vi "Rename.vi"() -> ()   [LabVIEW 2021]
uses:
  <vilib>/Utility/EditLVLibs/Edit LVLibs.lvlib
  _Rename/_Rename.lvlib
panel:
  in  "Name":string="Template"
  in  "Rename":bool
  in  "Rename":string="NEW"
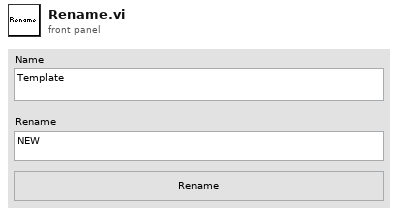
[diagram p1: front panel]
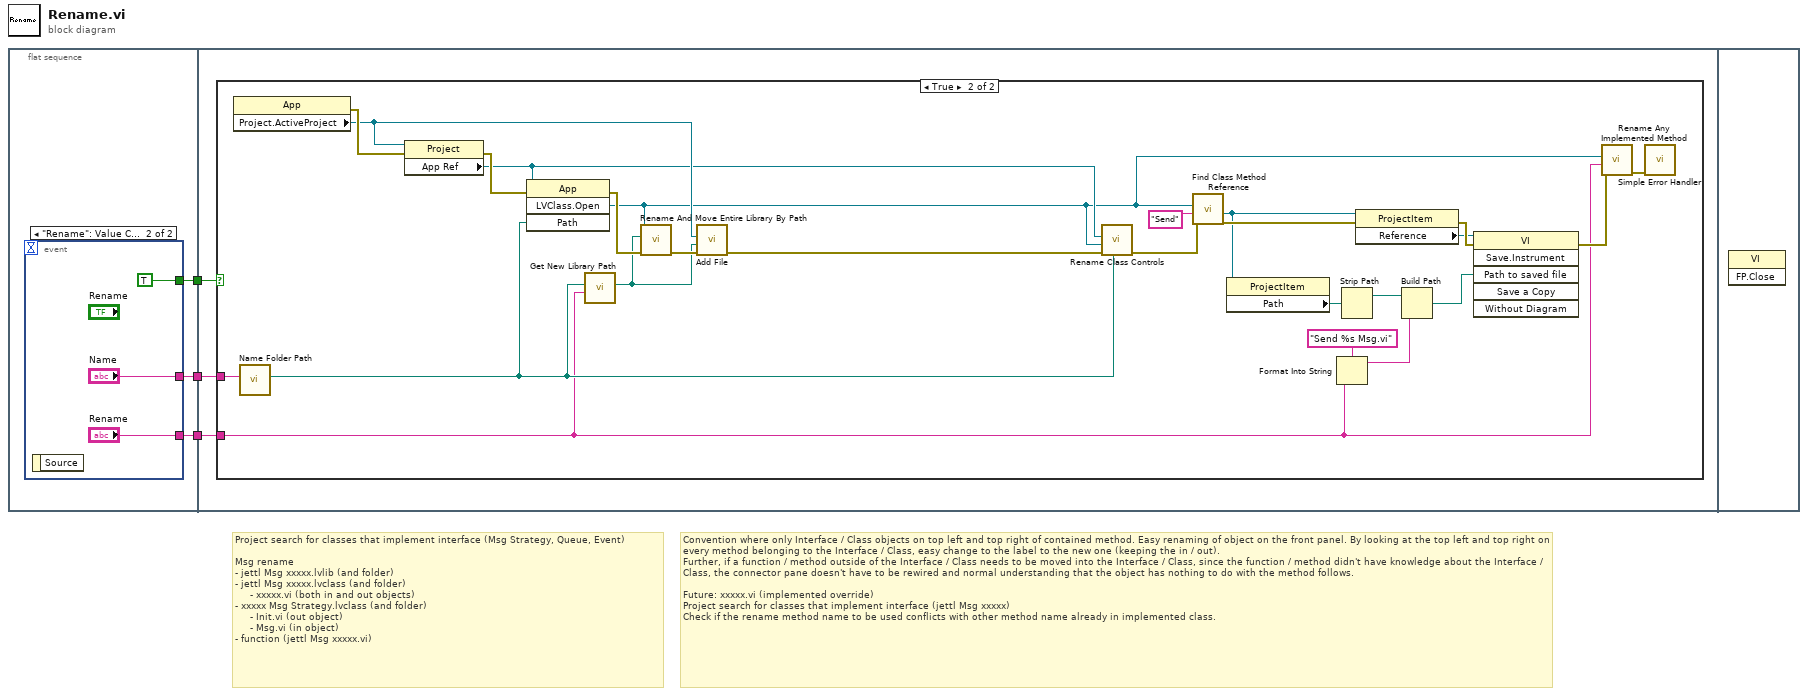
[diagram p0: block diagram]
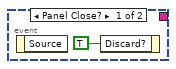
[diagram p2: hidden frame]
diagram:
  # "Convention where only Interface / Class objects on top left and top right of contained method. Easy renaming of object on the front panel. By looking at the top left and top right on every method belonging to the Interface / Class, easy change to the label to the new one (keeping the in / out).\nFurther, if a function / method outside of the Interface / Class needs to be moved into the Interface / Class, since the function / method didn't have knowledge about the Interface / Class, the connector pane doesn't have to be rewired and normal understanding that the object has nothing to do with the method follows.\n\nFuture: xxxxx.vi (implemented override)\nProject search for classes that implement interface (jettl Msg xxxxx)\nCheck if the rename method name to be used conflicts with other method name already in implemented class."
  # "Project search for classes that implement interface (Msg Strategy, Queue, Event)\n\nMsg rename\n- jettl Msg xxxxx.lvlib (and folder)\n- jettl Msg xxxxx.lvclass (and folder)\n     - xxxxx.vi (both in and out objects)\n- xxxxx Msg Strategy.lvclass (and folder)\n     - Init.vi (out object)\n     - Msg.vi (in object)\n- function (jettl Msg xxxxx.vi)"
  n1 = flat-sequence {
    tunnel: [w6] -> w3
    tunnel: [w5] -> w2
    tunnel: [w4] -> w1
    tunnel: w3 -> [w13]
    tunnel: w2 -> [w12]
    tunnel: w1 -> [w11]
    frame #0 {
      n2 = event shown="[1] \"Rename\": Value Change" {
        selector: _ -> [_ _]
        dyn-events: _ -> [_ _]
        timeout: _ -> [_ _]
        tunnel: [_ TRUE ("Rename 2")] -> w6
        tunnel: [_ "Rename"] -> w5
        tunnel: [_ "Name"] -> w4
        event Panel Close? {
          n3 = event-data() -> ()  [unwired: 1 in, 1 out]
          n4 = event-data("Discard?"=TRUE) -> ()  [unwired: 1 in, 1 out]
        }
        event "Rename": Value Change {
          n5 = event-data() -> ()  [unwired: 1 in, 1 out]
        }
      }
    }
    frame #1 {
      n6 = case shown="True" w13 {
        tunnel: w12 -> [_ w17]
        tunnel: w11 -> [_ w19]
        frame False {
        }
        frame True {
          n7 = property class="App"() -> (error out=w37:errorcluster, "Project.ActiveProject"=w21:refnum<vi>)  [unwired: 2 in, 1 out]
          n8 = call "Name Folder Path.vi"("Name"=w19) -> ("Name Folder Path"=w18:path)  [unwired: 10 in]
          n9 = property class="Project"(reference=w21, error in=w37) -> (error out=w35:errorcluster, "App Ref"=w20:refnum<vi>)  [unwired: 1 out]
          n10 = invoke class="App" method="LVClass.Open"(reference=w20, error in=w35, "Path"=w18) -> (error out=w36:errorcluster, "LVClass.Open"=w15:refnum<vi>)  [unwired: 1 in, 2 out]
          n11 = call "Get New Library Path.vi"("Rename"=w17, "Name Folder Path"=w18) -> ("New Library Path"=w16:path)  [unwired: 9 in]
          n12 = call <vilib>:"Rename And Move Entire Library By Path.vi"("error in (no error)"=w36, "New library path"=w16, "Library ref in"=w15) -> ("error out"=w22:errorcluster)  [unwired: 7 in, 1 out]
          n13 = call "Add File.vi"("error in"=w22, "Path"=w16, "Project:Active Project"=w21) -> ("error out"=w14:errorcluster)  [unwired: 8 in]
          n14 = call "Rename Class Controls.vi"("Old Class"=w18, "error in"=w14, "Class To Rename"=w15, "Application Instance"=w20) -> ("error out"=w27:errorcluster)  [unwired: 7 in]
          n15 = call "Find Class Method Reference.vi"("error in"=w27, "Method Name"="Send" ("regular expression"), "Class To Rename"=w15) -> ("error out"=w26:errorcluster, "Method Reference"=w23:refnum<vi>)  [unwired: 7 in]
          n16 = property class="ProjectItem"(reference=w23) -> ("Path"=w29:path)  [unwired: 1 in, 2 out]
          n17 = Format Into String(format string="Send %s Msg.vi", w17) -> (resulting string=w24:string)  [unwired: 2 in, 1 out]
          n18 = Strip Path(path=w29) -> (stripped path=w34:path)  [unwired: 1 out]
          n19 = property class="ProjectItem"(reference=w23, error in=w26) -> (error out=w38:errorcluster, "Reference"=w33:refnum<vi>)  [unwired: 1 out]
          n20 = Build Path(base path=w34, name or relative path=w24) -> (appended path=w32:path)
          n21 = invoke class="VI" method="Save.Instrument"(reference=w33, error in=w38, "Path to saved file"=w32) -> (error out=w30:errorcluster)  [unwired: 3 in, 5 out]
          n22 = call "Rename Any Implemented Method.vi"("error in"=w30, "Name"=w17, "Class To Rename"=w15) -> ("error out"=w31:errorcluster)  [unwired: 8 in]
          n23 = call <vilib>:"Simple Error Handler.vi"("error in (no error)"=w31) -> ()  [unwired: 4 in, 5 out]
        }
      }
    }
    frame #2 {
      n24 = invoke class="VI" method="FP.Close"() -> ()  [unwired: 3 in, 3 out]
    }
  }
